vi "Read Address.vi"(7 "Actor":refnum<class "Actor.lvclass">) -> (2 "Address":refnum<data-value>)   [LabVIEW 2025, in "jettl.lvlib" / "Transport.lvlib" / "Queue.lvlib"]
uses:
  Queue.lvlib
  Actor/Actor/Actor.lvclass
  Queue Transport/Queue Transport.lvclass
  Attributes/Attributes/Attributes.lvclass
  Msg/Msg.lvclass
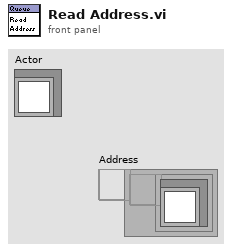
[diagram p1: front panel]
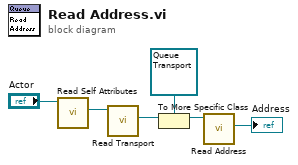
[diagram p0: block diagram]
diagram:
  n1 = call-dynamic "Read Self Attributes.vi"("Actor in"="Actor") -> ("Self Attributes"=w6:refnum<class "Attributes.lvclass">)  [unwired: 10 in]
  n2 = call-dynamic "Read Transport.vi"("Attributes in"=w6) -> ("Transport"=w5:refnum<class "Transport.lvclass">)  [unwired: 10 in]
  n3 = To More Specific Class(target class=refnum<class "Queue Transport.lvclass"> refnum ("jettl.lvlib:Transport.lvlib:Queue Transport.lvclass"), reference=w5) -> (specific class reference=w2:refnum<class "Queue Transport.lvclass">)  [unwired: 1 in, 1 out]
  n4 = call "Read Address.vi"("Queue Transport in"=w2) -> ("Address"=→"Address":refnum<data-value>)  [unwired: 10 in]
